vi "Data Type to String 1D.vi"(8 "error in (no error)":errorcluster, 11 "Data Type":refnum<class "Data Type.lvclass">) -> (0 "error out":errorcluster, 3 "String 1D out":string[](array[string]))   [LabVIEW 2017, in "String 1D.lvclass"]
uses:
  <vilib>/gpm_packages/@cs/data-type-serializer/source/String 1D/String 1D.lvclass
  <vilib>/gpm_packages/@cs/data-type-serializer/source/Data Type/Data Type.lvclass
  <vilib>/gpm_packages/@cs/data-type-serializer/source/String 1D/String 1D.lvclass/String 1D.ctl
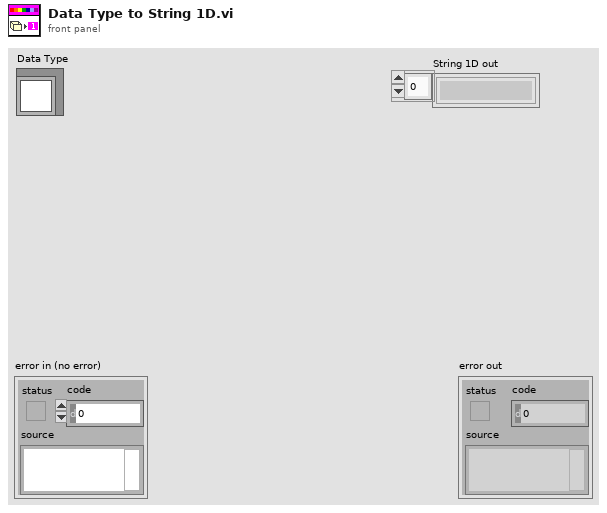
[diagram p1: front panel]
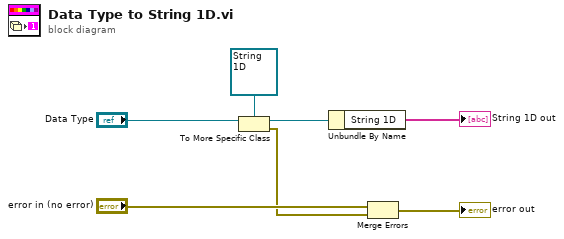
[diagram p0: block diagram]
diagram:
  n1 = To More Specific Class(target class=refnum<class "String 1D.lvclass"> refnum ("Boolean out"), reference="Data Type") -> (specific class reference=w4:refnum<class "String 1D.lvclass">, error out=w2:errorcluster)  [unwired: 1 in]
  n2 = Unbundle By Name(w4) -> ("String 1D"=→"String 1D out":string[])
  n3 = Merge Errors("error in (no error)", w2) -> (→"error out":errorcluster)
